vi "DHE_SetSizeVals.vi"(8 "error in":errorcluster, 9 "ytotsize":i32, 10 "xtotsize":i32) -> (0 "errorout":errorcluster)   [LabVIEW 2016]
uses:
  DBSHAND/private/vis/DatabaseHand_Element_Set(I32).vi
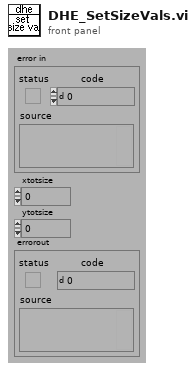
[diagram p1: front panel]
types:
  T1 = typedef "DatabaseHand_RefNum.ctl" = refnum<vi>
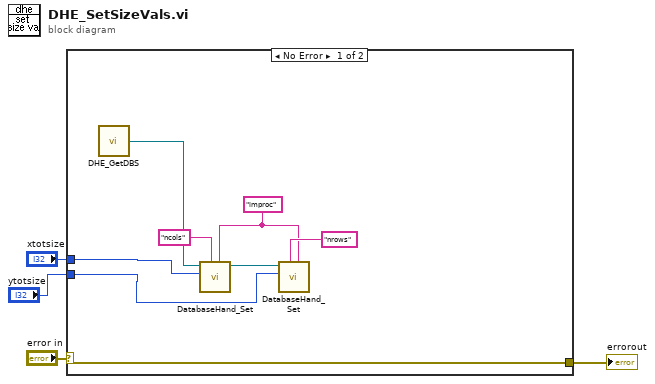
[diagram p0: block diagram]
diagram:
  n1 = case shown="No Error" "error in" {
    selector: "error in" -> [w12 w13]
    tunnel: "xtotsize" -> [w7 _]
    tunnel: "ytotsize" -> [w6 _]
    tunnel: [w12 w13] -> w1
    frame No Error {
      w9 = "improc" ("group")
      n2 = call "DHE_GetDBS.vi"() -> ("DHE_DBSRef"=w5:T1)  [unwired: 9 out]
      n3 = call-poly "DatabaseHand_Set.vi"("group"=w9, "name"="ncols", "value"=w7, "Database RefNum in"=w5) -> ("Database RefNum out"=w8:T1)  [unwired: 4 in, 3 out]
      n4 = call-poly "DatabaseHand_Set.vi"("group"=w9, "name"="nrows", "value"=w6, "Database RefNum in"=w8) -> ()  [unwired: 4 in, 4 out]
    }
    frame Error {
    }
  }
  "errorout" <- w1
